vi "Acquire.vi"(8 "error in (no error)":errorcluster, 10 "Msg in":T2, 11 "PXIDigitizer in":refnum<class "MagAnalysis_Online.lvclass">) -> (0 "error out":errorcluster, 1 "new command":string, 2 "Msg out":T2, 3 "PXIDigitizer out":refnum<class "MagAnalysis_Online.lvclass">)   [LabVIEW 2011, in "MagAnalysis_Online.lvclass"]
uses:
  MagAnalysis_Online.lvclass
  DriverMsg.ctl
  specInfo_TypDef.ctl
  specClustercommandTypdef.ctl
  reshapeArrayCommand_TypDEf.ctl
  MagAnalysis_Online.lvclass/MagAnalysis_Online.ctl
  BaseDriver/BaseDriver.lvclass
panel:
  out "time:FGV":u32
  out "time:updateSpec":u32
  out "time 2Dimage":u32
  out "time:specPost":u32
  out "time:div":u32
  out "time post":u32
  out "tima: aqu":u32
  out "offset":dbl
  in  "B [T] 2":dbl
  out "post":dbl[][](array[numeric])
  out "new ROI":bool
  in  "increment":bool
  out "online":dbl[][](array[numeric])
  out "cHARGE":dbl[][](array[numeric])
  out "time 3":u32
  out "time 2":u32
  out "time 1":u32
  out "time 0":u32
  out "time all":u32
  out "time get images":u32
  out "B [T]":dbl
  out "specInfo":T1 {"Charge [pC]" format="%0.4f"}
  in  "Numeric":i32=95
  out "Subscription OK":bool[](array[boolean])
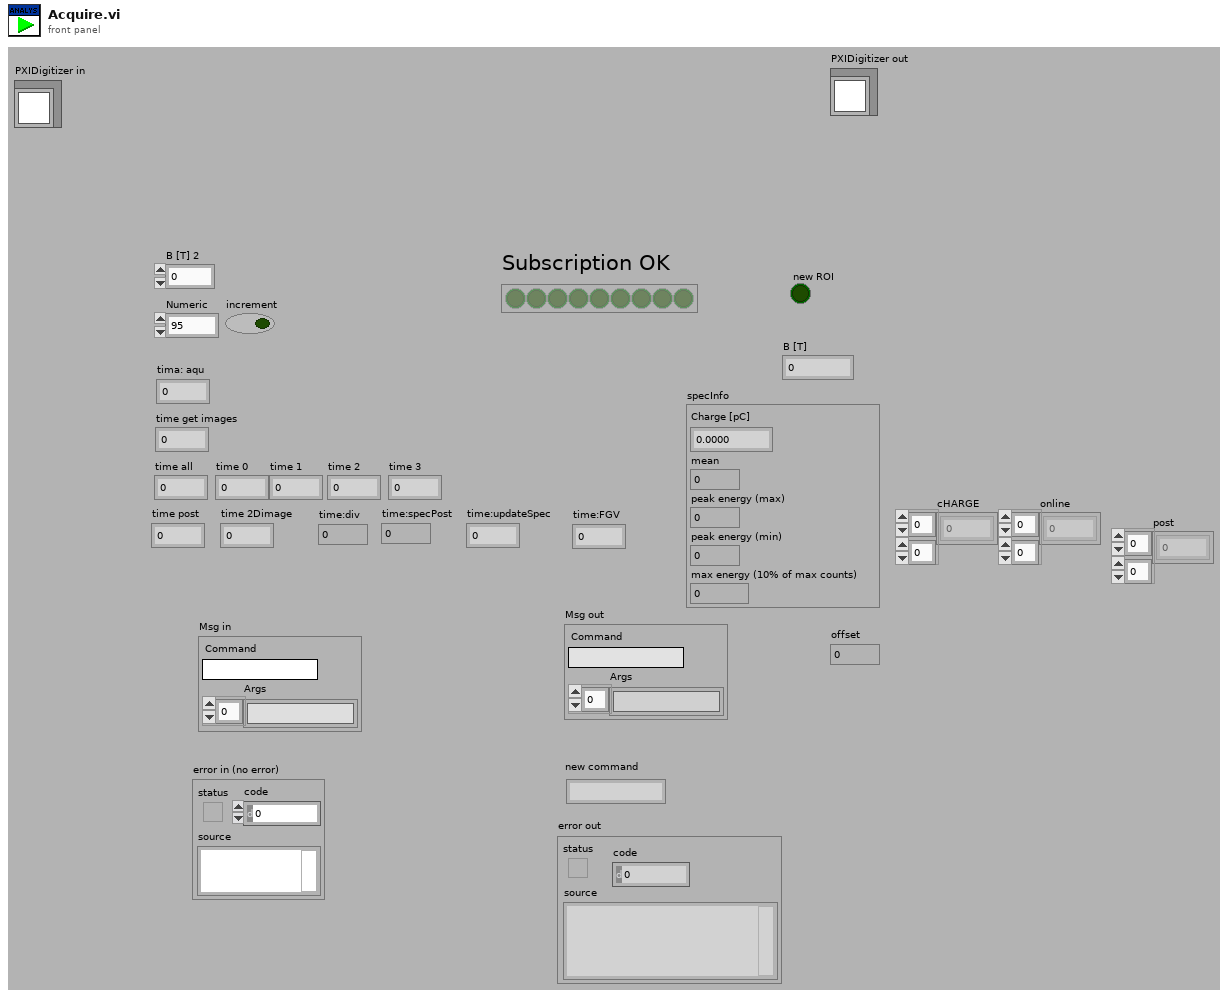
[diagram p1: front panel]
types:
  T1 = typedef "specInfo_TypDef.ctl" = cluster{"Charge [pC]":dbl, "mean":dbl, "peak energy (max)":dbl, "peak energy (min)":dbl, "max energy (10% of max counts)":dbl}
  T2 = typedef "DriverMsg.ctl" = cluster{"Command":string, "Args":string[]}
  T3 = typedef "reshapeArrayCommand_TypDEf.ctl" = enum16{"init array", "addImage", "read", "init resolution"}
  T4 = typedef "specClustercommandTypdef.ctl" = enum16{"init", "addCluster", "read"}
  T5 = typedef "fileCluster_TypDef.ctl" = cluster{"spec cluster":cluster{dbl[], dbl[]}, "change from file":dbl, "B [T]":dbl, "spec cluster 2":cluster{dbl[], dbl[]}[]}
  T6 = typedef "Calib_Typdef.ctl" = cluster{"cam 0":T7, "cam 1":T7, "cam 2":T7, "cam 3":T7}
  T7 = typedef "calib_Sub_Typdef.ctl" = cluster{"incident ANGLE COMPENSATION":dbl[], "field of view /pixel":dbl, "dp/B [MeV/C/B]":dbl[], "charge compensation":dbl[], "Momentum [MeV/C]":dbl[], "B [T]":dbl, "energyDependence Input":dbl[], "pixel angle (y)":dbl[], "dp [MeV/C/] ":dbl[], "angle 2Dfor spectrumj":dbl[][], "dp [MeV/C] 2D":dbl[][], "charge compensation 2D":dbl[][], "Screen&Camera 2":T8, "ROI info":T10, "Y 2D full angle":dbl[][]}
  T8 = typedef "ScreenCam2_TypDEf.ctl" = cluster{"Screen Orientation":string, "Screen angle":string, "Lens":T9, "Calibration (mm/pix)":dbl}
  T9 = typedef "CamAndObj_TypDEf.ctl" = enum16{"FL1-f8x08", "FL1-f8x06", "FL1-f8", "ch300-f50", "FL2G-f8", "FL3M14-f8", "FL3M14-f8x08", "FL3M14-f8x08(2x2)"}
  T10 = typedef "ROIInfo_TypDef.ctl" = cluster{"npix-X":i32, "npix-Y":i32, "Left [pix]":dbl, "Top [pix]":dbl}
  T11 = typedef "OnOffTypeDef.ctl" = enum16{"off", "on"}
  T12 = typedef "specCluster_Typdef.ctl" = cluster{"dp [MeV/C]":dbl[], dbl[]}
  T13 = typedef "IMAQ Image.ctl" = refnum<image>
  T14 = typedef "reshapeINfo_TypDef.ctl" = cluster{"emptyImageArray":dbl[], "max Y size":i32, "X size":i32, "min Y for allImage":dbl, "number of cam":i32, "emptyZArrayforreshape":T15}
  T15 = typedef "emptyArray_TYpDEf.ctl" = cluster{"Cam 0":T16, "Cam 1":T16, "Cam 2":T16, "Cam 3":T16}
  T16 = typedef "emptyArrayCamX_TypDef.ctl" = cluster{"1":dbl[][], "2":dbl[][]}
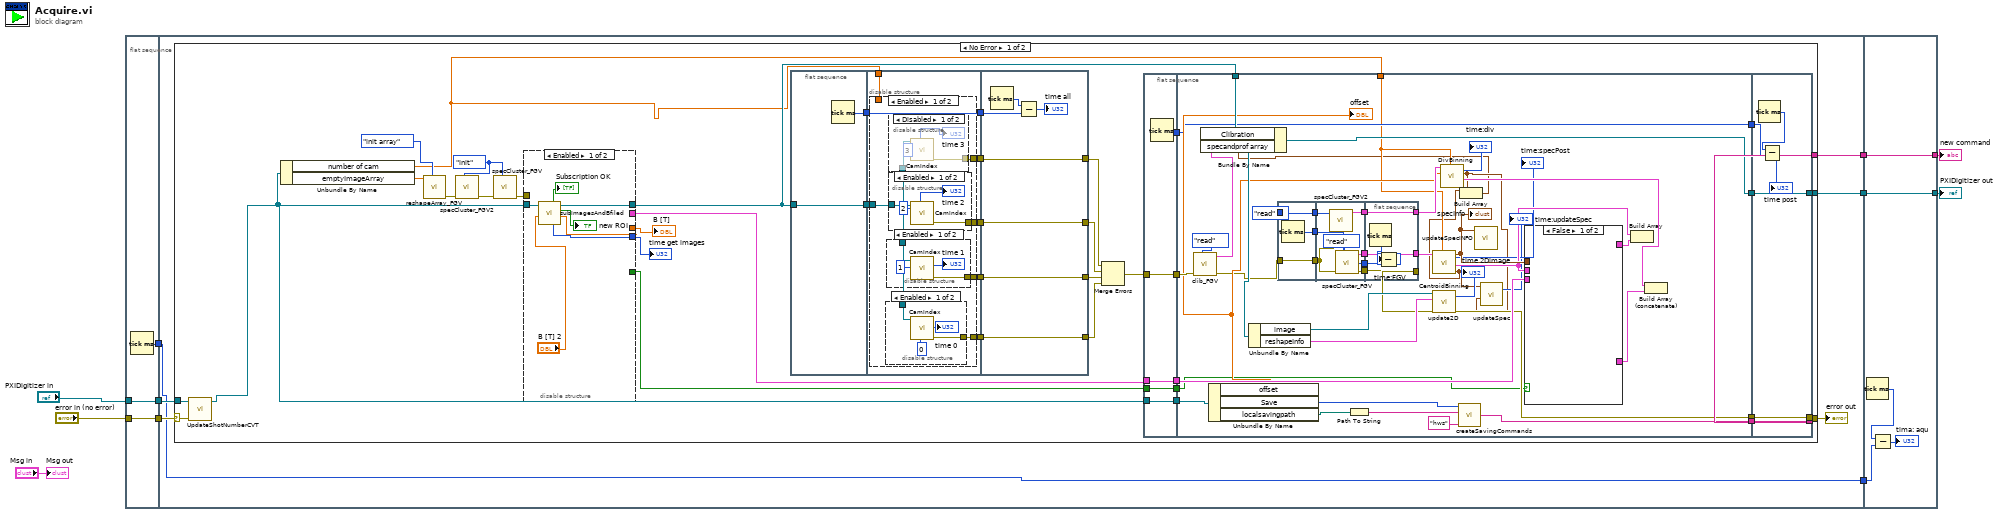
[diagram p0: block diagram]
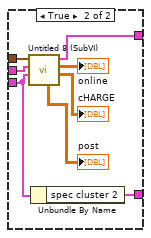
[diagram p2: hidden frame]
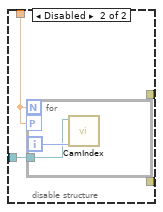
[diagram p7: hidden frame]
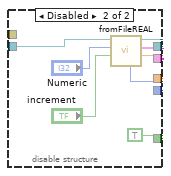
[diagram p8: hidden frame]
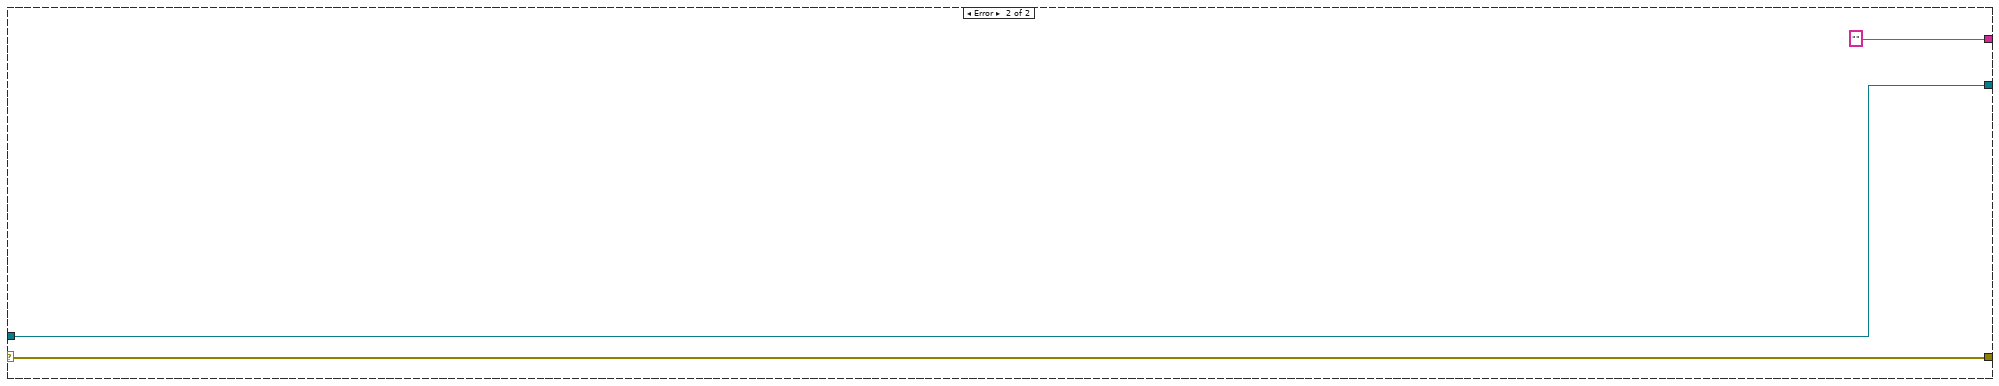
[diagram p9: hidden frame]
diagram:
  n1 = flat-sequence {
    tunnel: "error in (no error)" -> [w13]
    tunnel: "PXIDigitizer in" -> [w14]
    tunnel: [w14] -> w4
    tunnel: [w13] -> w3
    tunnel: [w12] -> w2
    tunnel: [w20] -> w6
    tunnel: [w16] -> w5
    tunnel: w4 -> [w19]
    tunnel: w3 -> [w17]
    tunnel: w2 -> [w15]
    tunnel: [w15] -> w1
    tunnel: [w200] -> w7
    tunnel: [w201] -> w11
    tunnel: w6 -> [w201]
    tunnel: w5 -> [w200]
    tunnel: w1 -> [w198]
    frame #0 {
      n2 = Tick Count (ms)() -> (millisecond timer value=w12:u32)
    }
    frame #1 {
      n3 = case shown="No Error" w17 {
        selector: w17 -> [w59 w195]
        tunnel: w19 -> [w58 w196]
        tunnel: [w38 w196] -> w20
        tunnel: [w37 w195] -> w18
        tunnel: [w35 "" ("new command")] -> w16
        frame No Error {
          w32 = specClustercommandTypdef."init" ("command")
          n4 = call "UpdateShotNumberCVT.vi"("error in (no error)"=w59, "BaseDriver in"=w58) -> ("BaseDriver out"=w36:refnum<class "MagAnalysis_Online.lvclass">)  [unwired: 8 in, 1 out]
          n5 = Unbundle By Name(w36) -> ("number of cam"=w21:dbl, "emptyImageArray"=w57:dbl[])
          n6 = call "reshapeArray_FGV.vi"("command"=reshapeArrayCommand_TypDEf."init array", "emptyImageArray"=w57) -> ("error in (no error) 2"=w34:errorcluster)  [unwired: 8 in, 1 out]
          n7 = call "specCluster_FGV2.vi"("command"=w32, "error in (no error)"=w34) -> ("error out"=w33:errorcluster)  [unwired: 8 in, 1 out]
          n8 = call "specCluster_FGV.vi"("command"=w32, "error in (no error)"=w33) -> ("error out"=w55:errorcluster)  [unwired: 8 in, 1 out]
          n9 = disable-structure shown="Enabled" {
            disable-tunnel: w55 -> [_ _]
            disable-tunnel: [w185 w193] -> w42
            disable-tunnel: [w184 w192] -> w22
            disable-tunnel: [w183 w187] -> w41
            disable-tunnel: w36 -> [w182 w189]
            disable-tunnel: [_ w188] -> w40
            disable-tunnel: [_ TRUE] -> w39
            frame Enabled {
              n10 = call "subImagesAndBfiled.vi"("B [T]"="B [T] 2", "MagAnalysis_Online in"=w182) -> ("B[T]"=w183:dbl, "new ROI"=→"new ROI":bool, "MagAnalysis_Online out"=w184:refnum<class "MagAnalysis_Online.lvclass">, "Numeric 2"=w185:u32, "OK"=→"Subscription OK":bool[])  [unwired: 5 in]
            }
            frame Disabled {
              n11 = call "fromFileREAL.vi"("increment"="increment", "Numeric"="Numeric", "MagAnalysis_Online in"=w189) -> ("B [T]"=w187:dbl, "Cluster"=w188:T5, "MagAnalysis_Online out"=w192:refnum<class "MagAnalysis_Online.lvclass">, "time"=w193:u32)  [unwired: 5 in]
            }
          }
          "B [T]" <- w41
          "time get images" <- w42
          n12 = flat-sequence {
            tunnel: w22 -> [w139]
            tunnel: [w139] -> w49
            tunnel: [w138] -> w44
            tunnel: w49 -> [w142]
            tunnel: [w146] -> w48
            tunnel: [w145] -> w47
            tunnel: [w144] -> w46
            tunnel: [w143] -> w45
            tunnel: w44 -> [w141]
            tunnel: [w141] -> w43
            tunnel: w21 -> [w140]
            tunnel: [w175] -> w51
            tunnel: [w176] -> w52
            tunnel: [w177] -> w53
            tunnel: [w178] -> w54
            tunnel: w48 -> [w178]
            tunnel: w47 -> [w177]
            tunnel: w46 -> [w176]
            tunnel: w45 -> [w175]
            tunnel: w43 -> [w173]
            frame #0 {
              n13 = Tick Count (ms)() -> (millisecond timer value=w138:u32)
            }
            frame #1 {
              n14 = disable-structure shown="Enabled" {
                disable-tunnel: [w151 _] -> w146
                disable-tunnel: [w150 _] -> w145
                disable-tunnel: [w149 _] -> w144
                disable-tunnel: [w148 _] -> w143
                disable-tunnel: w142 -> [w147 w169]
                disable-tunnel: w140 -> [_ w168]
                frame Enabled {
                  n15 = disable-structure shown="Enabled" {
                    disable-tunnel: [w167 _] -> w148
                    disable-tunnel: w147 -> [w166 _]
                    frame Enabled {
                      n16 = call "CamIndex.vi"("index"=0, "MagAnalysis_Online in"=w166) -> ("error out"=w167:errorcluster, "time"=→"time 0":u32)  [unwired: 5 in, 3 out]
                    }
                    frame Disabled {
                    }
                  }
                  n17 = disable-structure shown="Enabled" {
                    disable-tunnel: [w159 _] -> w149
                    disable-tunnel: w147 -> [w158 _]
                    frame Enabled {
                      n18 = call "CamIndex.vi"("index"=1, "MagAnalysis_Online in"=w158) -> ("error out"=w159:errorcluster, "time"=→"time 1":u32)  [unwired: 5 in, 3 out]
                    }
                    frame Disabled {
                    }
                  }
                  n19 = disable-structure shown="Enabled" {
                    disable-tunnel: [w155 _] -> w150
                    disable-tunnel: w147 -> [w154 _]
                    frame Enabled {
                      n20 = call "CamIndex.vi"("index"=2, "MagAnalysis_Online in"=w154) -> ("error out"=w155:errorcluster, "time"=→"time 2":u32)  [unwired: 5 in, 3 out]
                    }
                    frame Disabled {
                    }
                  }
                  n21 = disable-structure shown="Disabled" {
                    disable-tunnel: [w163 _] -> w151
                    disable-tunnel: w147 -> [w162 _]
                    frame Disabled {
                      n22 = call "CamIndex.vi"("index"=3, "MagAnalysis_Online in"=w162) -> ("error out"=w163:errorcluster, "time"=→"time 3":u32)  [unwired: 5 in, 3 out]
                    }
                    frame Enabled {
                    }
                  }
                }
                frame Disabled {
                  n23 = for {
                    N: w168 -> [_]
                    workers-P: w168 -> [_]
                    tunnel: w169 -> [w170]
                    i -> [w171]
                    n24 = call "CamIndex.vi"("index"=w171, "MagAnalysis_Online in"=w170) -> ()  [unwired: 5 in, 5 out]
                  }
                }
              }
            }
            frame #2 {
              n25 = Tick Count (ms)() -> (millisecond timer value=w174:u32)
              n26 = Subtract(x=w174, y=w173) -> (x-y=→"time all":u32)
            }
          }
          n27 = Merge Errors(w54, w53, w52, w51) -> (w50:errorcluster)
          n28 = flat-sequence {
            tunnel: w36 -> [w61]
            tunnel: w39 -> [w62]
            tunnel: w40 -> [w63]
            tunnel: w50 -> [w64]
            tunnel: [w64] -> w28
            tunnel: [w63] -> w27
            tunnel: [w62] -> w26
            tunnel: [w61] -> w25
            tunnel: [w60] -> w24
            tunnel: w22 -> [w99]
            tunnel: [w96] -> w31
            tunnel: [w95] -> w30
            tunnel: [w89] -> w29
            tunnel: w28 -> [w104]
            tunnel: w27 -> [w101]
            tunnel: w26 -> [w77]
            tunnel: w25 -> [w91]
            tunnel: w24 -> [w82]
            tunnel: [w82] -> w23
            tunnel: w21 -> [w68]
            tunnel: [w135] -> w35
            tunnel: [w136] -> w37
            tunnel: [w137] -> w38
            tunnel: w31 -> [w137]
            tunnel: w30 -> [w136]
            tunnel: w29 -> [w135]
            tunnel: w23 -> [w133]
            frame #0 {
              n29 = Tick Count (ms)() -> (millisecond timer value=w60:u32)
            }
            frame #1 {
              n30 = call "clib_FGV.vi"("command"=specClustercommandTypdef."read", "error in (no error)"=w104) -> ("error out"=w70:errorcluster, "Clibration 2"=w105:T6)  [unwired: 8 in]
              n31 = Unbundle By Name(w91) -> ("offset"=w83:dbl, "Save"=w90:T11, "localsavingpath"=w92:path)
              "offset" <- w83
              n32 = flat-sequence {
                tunnel: specClustercommandTypdef."read" ("command") -> [w110]
                tunnel: [w110] -> w73
                tunnel: [w109] -> w72
                tunnel: w70 -> [w108]
                tunnel: [w108] -> w69
                tunnel: [w116] -> w76
                tunnel: [w115] -> w75
                tunnel: [w113] -> w74
                tunnel: w73 -> [w114]
                tunnel: w72 -> [w112]
                tunnel: [w112] -> w71
                tunnel: w69 -> [w111]
                tunnel: [w121] -> w85
                tunnel: [w122] -> w87
                tunnel: [w123] -> w107
                tunnel: w76 -> [w123]
                tunnel: w75 -> [w122]
                tunnel: w74 -> [w121]
                tunnel: w71 -> [w119]
                frame #0 {
                  n33 = Tick Count (ms)() -> (millisecond timer value=w109:u32)
                }
                frame #1 {
                  n34 = call "specCluster_FGV2.vi"("command"=w114, "error in (no error)"=w111) -> ("specArray"=w113:T12[])  [unwired: 8 in, 1 out]
                  n35 = call "specCluster_FGV.vi"("command"=specClustercommandTypdef."read", "error in (no error)"=w111) -> ("error out"=w115:errorcluster, "specArray"=w116:T12[])  [unwired: 8 in]
                }
                frame #2 {
                  n36 = Tick Count (ms)() -> (millisecond timer value=w120:u32)
                  n37 = Subtract(x=w120, y=w119) -> (x-y=→"time:FGV":u32)
                }
              }
              n38 = Path To String(path=w92) -> (string=w93:string)
              n39 = call "CentroidBinning.vi"("Settings.number of cam"=w68, "spec cluster 3"=w107) -> ("spectrum"=w66:waveform(dbl), "spec cluster"=w102:cluster{"xi used":dbl[], "yi":dbl[]}, "specInfo"=w103:T1, "time:specPost"=→"time:specPost":u32)  [unwired: 5 in, 1 out]
              "specInfo" <- w103
              n40 = call "DivBinning.vi"("Settings.number of cam"=w68, "offset"=w83, "spec cluster 3"=w85) -> ("spec cluster"=w84:cluster{"xi used":dbl[], "yi":dbl[]}, "divergence"=w67:waveform(dbl), "time:div"=→"time:div":u32)  [unwired: 6 in]
              n41 = call "createSavingCommands.vi"("extension"="hws" ("Fileextension"), "Saving Path (local)"=w93, "Save"=w90) -> ("String"=w89:string)  [unwired: 1 in]
              n42 = Build Array(w66, w67) -> (w65:waveform(dbl)[])
              n43 = Bundle By Name(cluster=w99, "Clibration"=w105, "specandprof array"=w65) -> (w96:refnum<class "MagAnalysis_Online.lvclass">)
              n44 = Unbundle By Name(w96) -> ("image"=w98:T13, "reshapeInfo"=w97:T14)
              n45 = call "update2D.vi"("error in (no error)"=w87, "reshapeInfo"=w97, "Image in"=w98) -> ("error out"=w95:errorcluster, "time 2Dimage"=→"time 2Dimage":u32)  [unwired: 6 in, 1 out]
              n46 = call "updateSpecINFO.vi"("specInfo"=w103) -> ()  [unwired: 11 in]
              n47 = call "updateSpec.vi"("profile"=w67, "spectrum"=w66) -> ("time:updateSpec"=→"time:updateSpec":u32)  [unwired: 9 in]
              n48 = case shown="False" w77 {
                tunnel: w103 -> [_ w131]
                tunnel: w102 -> [_ w130]
                tunnel: w101 -> [_ w125]
                tunnel: [_ w129] -> w100
                tunnel: [_ w124] -> w88
                frame False {
                }
                frame True {
                  n49 = call "Untitled 8 (SubVI).vi"("Cluster 2"=w125, "spec cluster in"=w130, "specInfo"=w131) -> ("cHARGE"=→"cHARGE":dbl[][], "online"=→"online":dbl[][], "spec cluster out"=w129:cluster{dbl[], dbl[]}, "post"=→"post":dbl[][])  [unwired: 5 in]
                  n50 = Unbundle By Name(w125) -> ("spec cluster 2"=w124:cluster{dbl[], dbl[]}[])
                }
              }
              n51 = Build Array(w102, w100) -> ()  [unwired: 1 out]
              n52 = Build Array (concatenate)(w84, w88) -> ()  [unwired: 1 out]
            }
            frame #2 {
              n53 = Tick Count (ms)() -> (millisecond timer value=w134:u32)
              n54 = Subtract(x=w134, y=w133) -> (x-y=→"time post":u32)
            }
          }
        }
        frame Error {
        }
      }
      "error out" <- w18
    }
    frame #2 {
      n55 = Tick Count (ms)() -> (millisecond timer value=w199:u32)
      n56 = Subtract(x=w199, y=w198) -> (x-y=→"tima: aqu":u32)
    }
  }
  "PXIDigitizer out" <- w11
  "new command" <- w7
  "Msg out" <- "Msg in"
